vi "Query Lock In Amplifier Status.vi"(8 "error in (no error)":errorcluster, 11 "VISA resource name":refnum<visa-resource-name>) -> (0 "error out":errorcluster, 2 "Lock In Amplifier Data Message":string, 3 "VISA resource name out":refnum<visa-resource-name>)   [LabVIEW 2020, in "Stanford Research 830.lvlib"]
doc: "Queries the Lock-In Amplifier Status register for the Questionable Data Register group. Essentially, it is used to observe possible invalid results."
uses:
  Stanford Research 830.lvlib
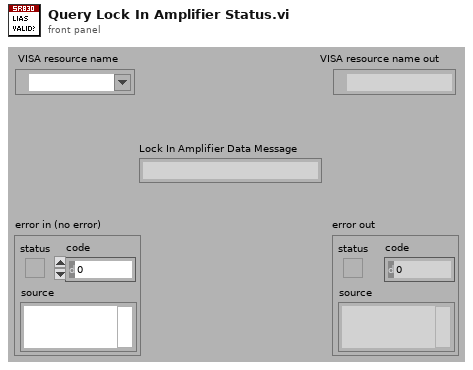
[diagram p1: front panel]
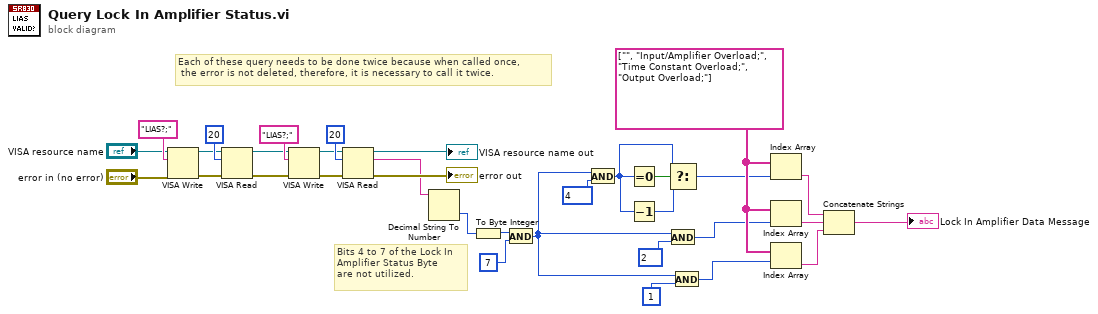
[diagram p0: block diagram]
diagram:
  w25 = string[] ["", "Input/Amplifier Overload;", "Time Constant Overload;", "Output Overload;"]
  # "Each of these query needs to be done twice because when called once,\n the error is not deleted, therefore, it is necessary to call it twice."
  # "Bits 4 to 7 of the Lock In \nAmplifier Status Byte \nare not utilized."
  n1 = VISA Write(VISA resource name="VISA resource name", write buffer="LIAS?;", error in (no error)="error in (no error)") -> (VISA resource name out=w30:refnum<visa-resource-name>, error out=w29:errorcluster)  [unwired: 1 out]
  n2 = VISA Read(VISA resource name=w30, byte count=u32 20, error in (no error)=w29) -> (VISA resource name out=w5:refnum<visa-resource-name>, error out=w4:errorcluster)  [unwired: 2 out]
  n3 = VISA Write(VISA resource name=w5, write buffer="LIAS?;", error in (no error)=w4) -> (VISA resource name out=w7:refnum<visa-resource-name>, error out=w6:errorcluster)  [unwired: 1 out]
  n4 = VISA Read(VISA resource name=w7, byte count=u32 20, error in (no error)=w6) -> (VISA resource name out=→"VISA resource name out":refnum<visa-resource-name>, read buffer=w1:string, error out=→"error out":errorcluster)  [unwired: 1 out]
  n5 = Decimal String To Number(string=w1) -> (number=w33:i32)  [unwired: 2 in, 1 out]
  n6 = To Byte Integer(number=w33) -> (8bit integer=w24:i8)
  n7 = And(x=w24, y=i8 7 ("value")) -> (x .and. y?=w10:i8)
  n8 = And(x=w10, y=i8 4) -> (x .and. y?=w14:i8)
  n9 = Equal To 0?(x=w14) -> (x = 0?=w19:bool)
  n10 = Decrement(x=w14) -> (x-1=w18:i8)
  n11 = Select(t=w14, s=w19, f=w18) -> (s? t:f=w17:i8)
  n12 = And(x=w10, y=i8 2) -> (x .and. y?=w16:i8)
  n13 = And(x=w10, y=i8 1) -> (x .and. y?=w15:i8)
  n14 = Index Array(array=w25, index=w17) -> (element=w20:string)
  n15 = Index Array(array=w25, index=w16) -> (element=w12:string)
  n16 = Index Array(array=w25, index=w15) -> (element=w11:string)
  n17 = Concatenate Strings(w20, w12, w11) -> (→"Lock In Amplifier Data Message":string)
